vi "Executing.vi"(8 "error in (no error)":errorcluster, 11 "Do Nothing Command in":refnum<class "Do Nothing Command.lvclass">) -> (0 "error out":errorcluster, 3 "Do Nothing Command out":refnum<class "Do Nothing Command.lvclass">)   [LabVIEW 2013, in "Receiver.lvlib" / "Receiver Commands using Actor.lvlib" / "Do Nothing Command.lvclass"]
uses:
  Do Nothing Command.lvclass
  Receiver Command.lvclass
  <vilib>/ActorFramework/Message Enqueuer/Message Enqueuer.lvclass/Message Enqueuer.ctl
  <vilib>/ActorFramework/Message Enqueuer/Enqueue.vi
  <vilib>/ActorFramework/Message Priority Queue/Priority Enqueue.vi
  Command Actor/Command States Messages/Go To Completing Command Msg/Go To Completing Command Msg.lvclass
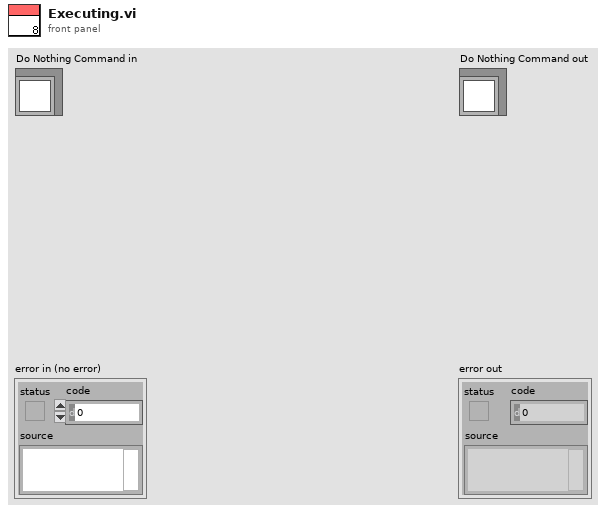
[diagram p1: front panel]
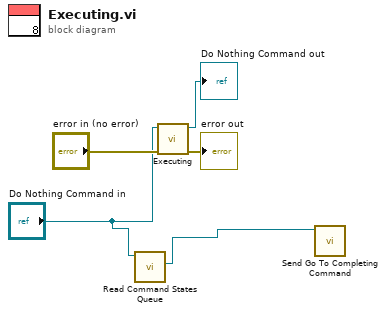
[diagram p0: block diagram]
diagram:
  n1 = call-dynamic "Read Command States Queue.vi"("Command Actor in"="Do Nothing Command in") -> ("Actor Framework:Message Enqueuer"=w1:refnum<class "Message Enqueuer.lvclass">)  [unwired: 8 in, 2 out]
  n2 = call-parent "Executing.vi"("error in (no error)"="error in (no error)", "Command Actor in"="Do Nothing Command in") -> ("error out"=→"error out":errorcluster, "Command Actor out"=→"Do Nothing Command out":refnum<class "Do Nothing Command.lvclass">)  [unwired: 8 in]
  n3 = call "Send Go To Completing Command.vi"("Message Enqueuer"=w1) -> ()  [unwired: 9 in, 2 out]
